vi "Handle SET.vi"(8 "error in (no error)":errorcluster, 10 "Param":variant, 11 "Instrument in":refnum<class "Instrument.lvclass">) -> (0 "error out":errorcluster, 2 "Data":variant, 3 "Instrument out":refnum<class "Instrument.lvclass">)   [LabVIEW 2019, in "Instrument.lvclass"]
uses:
  Instrument.lvclass
  Typedefs/Instrument.SET--cluster.ctl
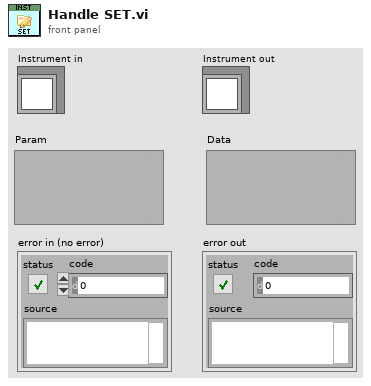
[diagram p1: front panel]
types:
  T1 = typedef "Instrument.lvclass/Instrument.SET--cluster.ctl" = cluster{"parameter":string, "Data":variant}
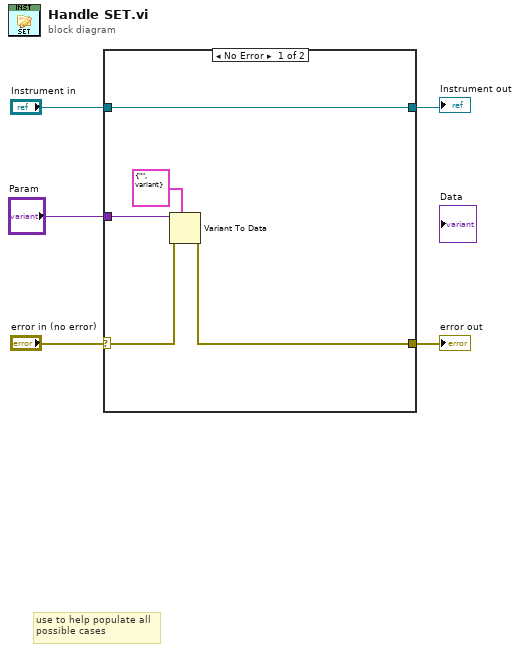
[diagram p0: block diagram]
diagram:
  # "use to help populate all\npossible cases"
  n1 = case shown="No Error" "error in (no error)" {
    selector: "error in (no error)" -> [w7 w11]
    tunnel: [w10 w12] -> w5
    tunnel: "Instrument in" -> [w10 w12]
    tunnel: [w6 w11] -> w3
    tunnel: "Param" -> [w8 _]
    frame No Error {
      n2 = Variant To Data(error in=w7, type=T1 {"parameter"="", "Data"=variant} ("GETSET"), Variant=w8) -> (error out=w6:errorcluster)  [unwired: 1 out]
    }
    frame Error {
    }
  }
  "Instrument out" <- w5
  "error out" <- w3
